vi "getMagnet.vi"(6 "Axis":T1, 8 "error in (no error)":errorcluster, 11 "Instrument.Cryostat in":refnum<class "Instrument.Cryostat.lvclass">) -> (0 "error out":errorcluster, 1 "Status":string, 2 "B Field (T)":dbl, 3 "Instrument.Cryostat out":refnum<class "Instrument.Cryostat.lvclass">, 4 "Finished?":bool)   [LabVIEW 2019, in "Instrument.Cryostat.lvclass"]
uses:
  Instrument.Cryostat.lvclass
  C:/Users/patrick/Documents/GitHub/Instrument-Framework/lvsrc/Instrument/Instrument.lvclass
  Typedefs/Magnet Axis--Enum.ctl
  Typedefs/getMagnet--cluster.ctl
  Instrument/Instrument.lvclass/Instrument.ctl
  d99fca9a-0ec4-4724-b19e-b90548b9cfa0.vi
  d99fca9a-0ec4-4724-b19e-b90548b9cfa0.vi/fd31576d-e45a-45e4-abf0-bb66ac4deaa1.vi
  Instrument/API/Send and Receive.vi
  d99fca9a-0ec4-4724-b19e-b90548b9cfa0.vi/8ac3cdd8-092d-4e77-a3e0-d6c398d573f0.vi
  Instrument/Private/Get Client Type.vi
  d99fca9a-0ec4-4724-b19e-b90548b9cfa0.vi/fd31576d-e45a-45e4-abf0-bb66ac4deaa1.vi/f91c6170-9513-44c8-baa5-1ae8a5a1c276.vi
  d99fca9a-0ec4-4724-b19e-b90548b9cfa0.vi/fd31576d-e45a-45e4-abf0-bb66ac4deaa1.vi/28df1783-be57-4f54-a06b-ef948bbb2c31.vi
  d99fca9a-0ec4-4724-b19e-b90548b9cfa0.vi/8ac3cdd8-092d-4e77-a3e0-d6c398d573f0.vi/0ff7dfe4-58e3-4701-b078-d20c6dfb2558.vi
  d99fca9a-0ec4-4724-b19e-b90548b9cfa0.vi/8ac3cdd8-092d-4e77-a3e0-d6c398d573f0.vi/0be26b56-a647-41a0-b030-07ba82a41275.vi
  d99fca9a-0ec4-4724-b19e-b90548b9cfa0.vi/8ac3cdd8-092d-4e77-a3e0-d6c398d573f0.vi/0ff7dfe4-58e3-4701-b078-d20c6dfb2558.vi/8b8460ad-5430-459a-bed8-bcae5e64dc62.vi
  d99fca9a-0ec4-4724-b19e-b90548b9cfa0.vi/8ac3cdd8-092d-4e77-a3e0-d6c398d573f0.vi/0ff7dfe4-58e3-4701-b078-d20c6dfb2558.vi/cd230499-84e6-4a66-af6f-308924170b0e.vi
  Instrument/Private/Get RC Connection Status.vi
  Instrument/API/Enum to String.vi
  <userlib>/LevyLab/RemoteControl/API/Send and Receive.vi
  <vilib>/Utility/Data Type/Get Type Information.vi
  <vilib>/JDP Science/JSONtext/JSON text to Variant.vi
  Instrument/API/Instrument.GetPublicEvents.vi
  <vilib>/JDP Science/JSONtext/Variant to JSON Text.vi
  <vilib>/National Instruments/GUID Generator/Guid Generator.vi
  Instrument/API/Instrument.sendMessageToProcess.vi
  Instrument/Private/Instrument.MessageFromProcess.EventStructure.vi
  <vilib>/JDP Science/JSONtext/LVClass Serializer/JSONtext LVClass Serializer.lvclass
  Instrument/Instrument.lvclass
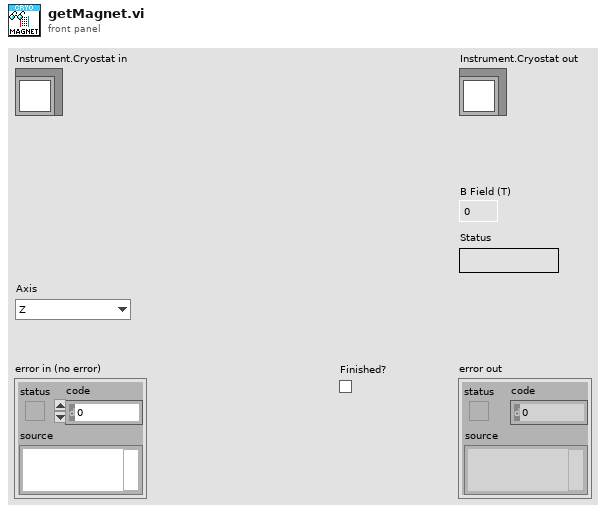
[diagram p1: front panel]
types:
  T1 = typedef "Instrument.Cryostat.lvclass/Magnet Axis--Enum.ctl" = enum16{"Z", "X", "Y"}
  T2 = typedef "Instrument.Cryostat.lvclass/getMagnet--cluster.ctl" = cluster{"Field (T)":dbl, "Status":string, "Finished?":bool}
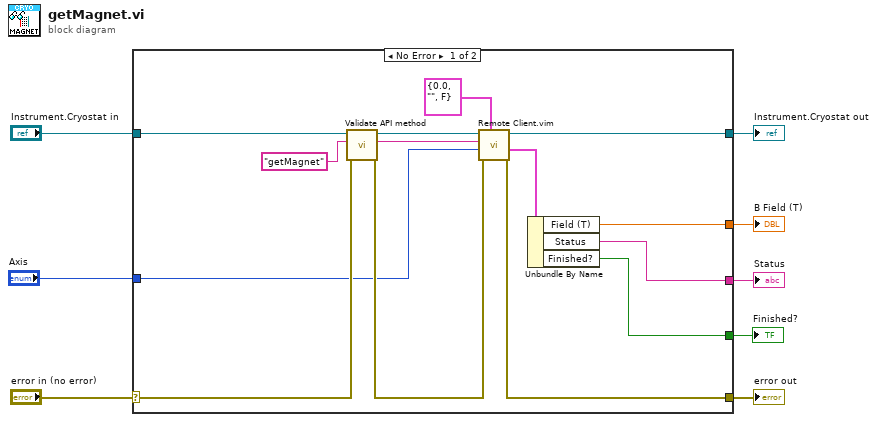
[diagram p0: block diagram]
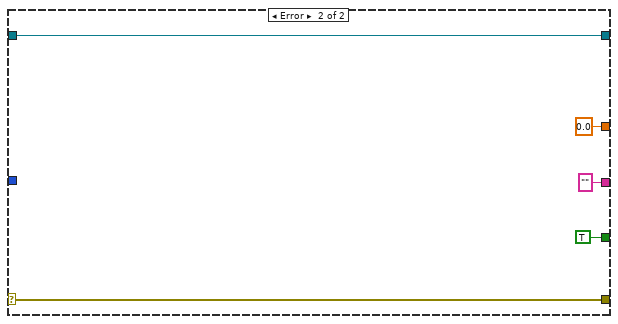
[diagram p2: hidden frame]
diagram:
  n1 = case shown="No Error" "error in (no error)" {
    selector: "error in (no error)" -> [w18 w27]
    tunnel: [w16 w27] -> w7
    tunnel: [w15 w26] -> w5
    tunnel: "Instrument.Cryostat in" -> [w19 w26]
    tunnel: "Axis" -> [w14 _]
    tunnel: [w11 0.0 ("Field (T)")] -> w3
    tunnel: [w10 "" ("Status")] -> w2
    tunnel: [w9 TRUE] -> w1
    frame No Error {
      n2 = call "Validate API method.vi"("error in (no error)"=w18, "command in"="getMagnet" ("error message (\"\")"), "Instrument in"=w19) -> ("error out"=w17:errorcluster, "command out"=w21:string, "Instrument out"=w20:refnum<class "Instrument.Cryostat.lvclass">)  [unwired: 6 in]
      n3 = call "Remote Client.vim"("Data Out type"=T2 {"Field (T)"=0.0, "Status"="", "Finished?"=FALSE} ("getMagnet"), "error in (no error)"=w17, "params"=w14, "method"=w21, "Instrument in"=w20) -> ("error out"=w16:errorcluster, "Data out"=w12:T2, "Instrument out"=w15:refnum<class "Instrument.Cryostat.lvclass">)  [unwired: 3 in, 1 out]
      n4 = Unbundle By Name(w12) -> ("Field (T)"=w11:dbl, "Status"=w10:string, "Finished?"=w9:bool)
    }
    frame Error {
    }
  }
  "error out" <- w7
  "Instrument.Cryostat out" <- w5
  "B Field (T)" <- w3
  "Status" <- w2
  "Finished?" <- w1
